vi "Select Role.vi"(8 "error in (no error)":errorcluster, 10 "Select Role":string, 11 "Roles API in":refnum<class "Roles API.lvclass">) -> (0 "error out":errorcluster, 3 "Roles API out":refnum<class "Roles API.lvclass">)   [LabVIEW 2020, in "Volatus.lvlib" / "Roles API.lvclass"]
uses:
  Roles API.lvclass
  Roles API.lvclass/Roles API.ctl
  MessageQ/MessageQ.lvclass
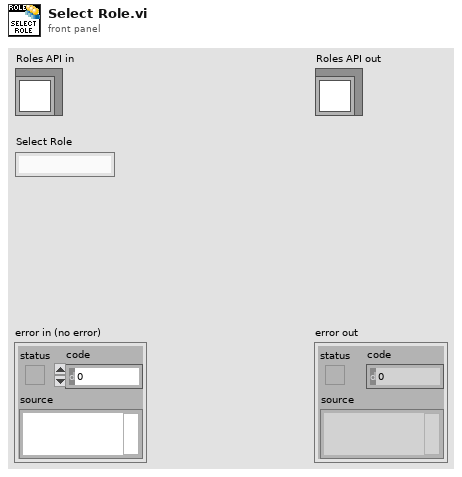
[diagram p1: front panel]
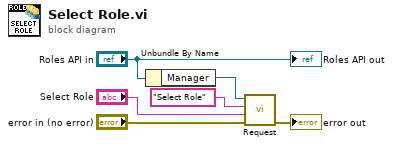
[diagram p0: block diagram]
diagram:
  n1 = Unbundle By Name("Roles API in") -> ("Manager"=w5:refnum<class "MessageQ.lvclass">)
  n2 = call "Request.vi"("error in (no error)"="error in (no error)", "Data"="Select Role", "ID"="Select Role", "MessageQ in"=w5) -> ("error out"=→"error out":errorcluster)  [unwired: 5 in, 2 out]
  "Roles API out" <- "Roles API in"
